vi "myRIO v1.0 Close AudioOut Block.vi"(7 "Scaling Constants List":T1, 8 "error in (no error)":errorcluster, 10 "AudioOut (N Samples) Channel List":T5, 11 "myRIO Ref In":T3) -> (0 "error out":errorcluster)   [LabVIEW 2021]
uses:
  <vilib>/myRIO/Common/Instrument Driver Framework/myRIO v1.0/AudioOut Block/typedefs/AudioOut Block Channels List.ctl
  <vilib>/myRIO/Common/Instrument Driver Framework/myRIO v1.0/AudioOut Block/typedefs/AudioOut Block Channels Enum.ctl
  <vilib>/myRIO/Common/Instrument Driver Framework/Utilities/typedefs/myRIO v1.0 Reference.ctl
  <vilib>/myRIO/Common/Instrument Driver Framework/Utilities/typedefs/Generic FPGA Reference.ctl
  <vilib>/myRIO/Common/Instrument Driver Framework/Utilities/typedefs/Analog Scaling Constants List.ctl
  <vilib>/myRIO/Common/Instrument Driver Framework/Utilities/typedefs/Analog Scaling Constants.ctl
  <vilib>/myRIO/Common/Instrument Driver Framework/myRIO v1.0/Resource Manager/vis/myRIO v1.0 Unreserve Channel List.vi
  <vilib>/myRIO/Common/Instrument Driver Framework/myRIO v1.0/AudioOut Block/vis/myRIO v1.0 Build MUX Configuration AudioOut Block.vi
  <vilib>/myRIO/Common/Instrument Driver Framework/myRIO v1.0/Resource Manager/vis/myRIO v1.0 Unreserve Channel.vi
  <vilib>/myRIO/Common/Instrument Driver Framework/myRIO v1.0/Resource Manager/vis/myRIO v1.0 Build Mutex Name.vi
  <vilib>/myRIO/Common/Instrument Driver Framework/myRIO v1.0/Resource Manager/vis/myRIO v1.0 Block Write Resource Manager.vi
  <vilib>/myRIO/Common/Instrument Driver Framework/myRIO v1.0/Resource Manager/vis/myRIO v1.0 Block Write Counter.vi
  <vilib>/myRIO/Common/Instrument Driver Framework/Utilities/vis/Configuration Manager.vi
  <vilib>/myRIO/Common/Instrument Driver Framework/Utilities/vis/IO Manager.vi
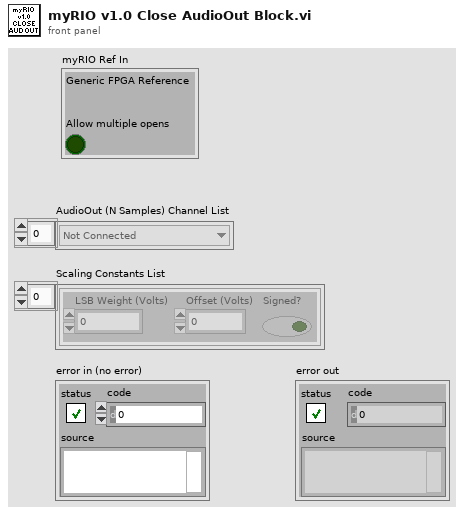
[diagram p1: front panel]
types:
  T1 = typedef "Analog Scaling Constants List.ctl" = T2[]
  T2 = typedef "Analog Scaling Constants.ctl" = cluster{"LSB Weight (Volts)":dbl, "Offset (Volts)":dbl, "Signed?":bool}
  T3 = typedef "myRIO v1.0 Reference.ctl" = cluster{"Generic FPGA Reference":T4, "Allow multiple opens":bool}
  T4 = typedef "Generic FPGA Reference.ctl" = refnum<k20>
  T5 = typedef "AudioOut Block Channels List.ctl" = T6[]
  T6 = typedef "AudioOut Block Channels Enum.ctl" = enum16{"Not Connected", "AudioOut/Left (N Samples)", "AudioOut/Right (N Samples)"}
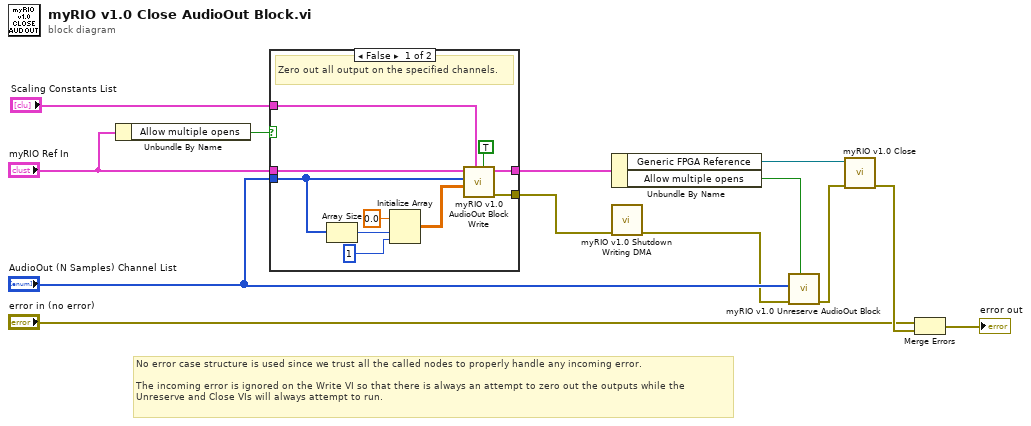
[diagram p0: block diagram]
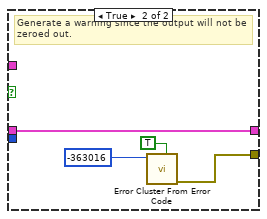
[diagram p2: hidden frame]
diagram:
  # "No error case structure is used since we trust all the called nodes to properly handle any incoming error.\n\nThe incoming error is ignored on the Write VI so that there is always an attempt to zero out the outputs while the Unreserve and Close VIs will always attempt to run."
  n1 = Unbundle By Name("myRIO Ref In") -> ("Allow multiple opens"=w7:bool)
  n2 = case shown="False" w7 {
    tunnel: "AudioOut (N Samples) Channel List" -> [w20 _]
    tunnel: "myRIO Ref In" -> [w22 w26]
    tunnel: [w18 w26] -> w11
    tunnel: [w17 w27] -> w2
    tunnel: "Scaling Constants List" -> [w19 _]
    frame False {
      # "Zero out all output on the specified channels."
      n3 = Array Size(array=w20) -> (size(s)=w16:i32)
      n4 = Initialize Array(0.0 ("element"), w16, 1 ("dimension size")) -> (w21:dbl[][])
      n5 = call <vilib>:"myRIO v1.0 AudioOut Block Write.vi"("Wait Until Done?"=TRUE, "Scale Constants Array"=w19, "dbl Scaled Value List"=w21, "AudioOut (N Samples) Channel List"=w20, "myRIO Ref In"=w22) -> ("error out"=w17:errorcluster, "myRIO Ref Out"=w18:T3)  [unwired: 5 in]
    }
    frame True {
      # "Generate a warning since the output will not be zeroed out."
      n6 = call <vilib>:"Error Cluster From Error Code.vi"("is warning? (False)"=TRUE, "error code (0)"=-363016) -> ("error out"=w27:errorcluster)  [unwired: 7 in]
    }
  }
  n7 = Unbundle By Name(w11) -> ("Generic FPGA Reference"=w4:T4, "Allow multiple opens"=w6:bool)
  n8 = call <vilib>:"myRIO v1.0 Shutdown Writing DMA.vi"("error in (no error)"=w2) -> ("error out"=w1:errorcluster)  [unwired: 10 in]
  n9 = call <vilib>:"myRIO v1.0 Unreserve AudioOut Block.vi"("Allow multiple opens?"=w6, "error in (no error)"=w1, "AudioOut (N Samples) Channel List"="AudioOut (N Samples) Channel List") -> ("error out"=w10:errorcluster)  [unwired: 8 in]
  n10 = call <vilib>:"myRIO v1.0 Close.vi"("error in (no error)"=w10, "myRIO FPGA Ref In"=w4) -> ("error out"=w9:errorcluster)  [unwired: 9 in]
  n11 = Merge Errors("error in (no error)", w9) -> (→"error out":errorcluster)
